vi "calc_rms.vi"(6 "Sampling Frequency [Hz]":dbl, 11 "Voltage [V]":dbl[](array[numeric])) -> (2 "Detected Frequency [Hz":dbl, 3 "RMS [V]":dbl)   [LabVIEW 2025, in "LabJackEKG.lvlib"]
uses:
  LabJackEKG.lvlib
  <vilib>/Analysis/2dsp.llb/Real FFT.vi
  <vilib>/Analysis/NI_AALPro.lvlib
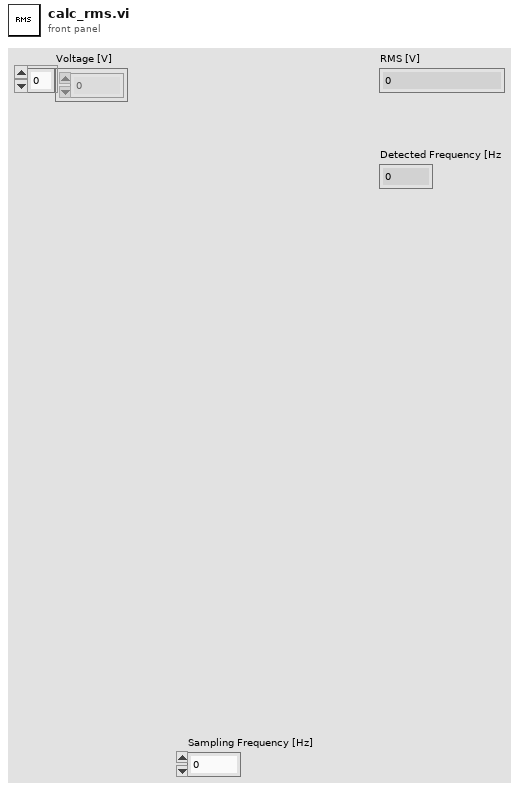
[diagram p1: front panel]
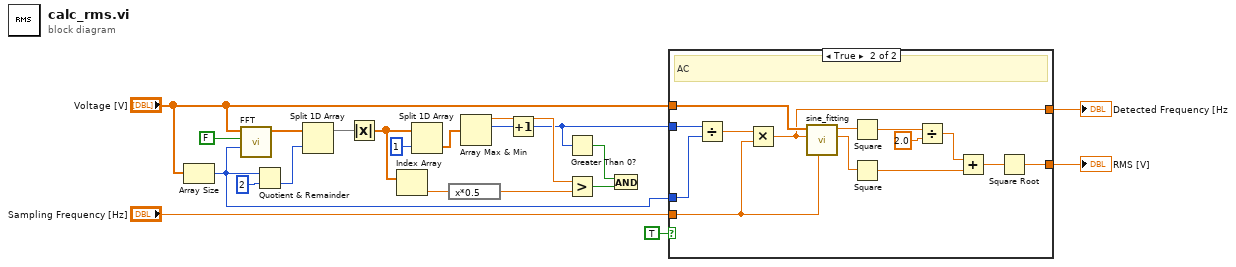
[diagram p0: block diagram]
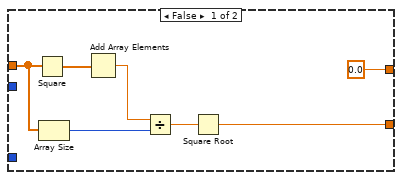
[diagram p2: hidden frame]
diagram:
  n1 = Array Size(array="Voltage [V]") -> (size(s)=w16:i32)
  n2 = call-poly <vilib>:"FFT.vi"("FFT size"=w16, "shift?"=FALSE, "X"="Voltage [V]") -> ("FFT {X}"=w8:cdb[])  [unwired: 7 in, 1 out]
  n3 = Quotient & Remainder(x=w16, y=2) -> (floor(x/y)=w10:i32)  [unwired: 1 out]
  n4 = Split 1D Array(array=w8, index=w10) -> (first subarray=w9:cdb[])  [unwired: 1 out]
  n5 = Absolute Value(x=w9) -> (abs(x)=w11:dbl[])
  n6 = Index Array(array=w11) -> (element=w13:dbl)  [unwired: 1 in]
  n7 = Split 1D Array(array=w11, index=1) -> (second subarray=w3:dbl[])  [unwired: 1 out]
  n8 = expression code="x*0.5"(w13) -> (w14:dbl)
  n9 = Array Max & Min(array=w3) -> (max value=w12:dbl, max index (indices)=w4:i32)  [unwired: 2 out]
  n10 = Increment(x=w4) -> (x+1=w1:i32)
  n11 = Greater Than 0?(x=w1) -> (x > 0?=w21:bool)
  n12 = Greater?(x=w12, y=w14) -> (0:w20:bool)
  n13 = And(x=w21, y=w20) -> ()  [unwired: 1 out]
  n14 = case shown="True" TRUE {
    tunnel: "Sampling Frequency [Hz]" -> [_ w38]
    tunnel: "Voltage [V]" -> [w24 w42]
    tunnel: w1 -> [_ w41]
    tunnel: w16 -> [_ w40]
    tunnel: [w25 w32] -> w17
    tunnel: [0.0 w29] -> w18
    frame False {
      n15 = Square(x=w24) -> (x^2=w28:dbl[])
      n16 = Array Size(array=w24) -> (size(s)=w23:i32)
      n17 = Add Array Elements(numeric array=w28) -> (sum=w27:dbl)
      n18 = Divide(x=w27, y=w23) -> (x/y=w26:dbl)
      n19 = Square Root(x=w26) -> (sqrt(x)=w25:dbl)
    }
    frame True {
      # "AC"
      n20 = Divide(x=w41, y=w40) -> (x/y=w39:dbl)
      n21 = Multiply(x=w39, y=w38) -> (x*y=w29:dbl)
      n22 = call "sine_fitting.vi"("Sampling Frequency [Hz]"=w38, "Frequency [Hz]"=w29, "RX data"=w42) -> ("DC Offset"=w36:dbl, "Amplidude"=w37:dbl)  [unwired: 7 in]
      n23 = Square(x=w37) -> (x^2=w34:dbl)
      n24 = Square(x=w36) -> (x^2=w30:dbl)
      n25 = Divide(x=w34, y=2.0) -> (x/y=w31:dbl)
      n26 = Add(x=w31, y=w30) -> (x+y=w33:dbl)
      n27 = Square Root(x=w33) -> (sqrt(x)=w32:dbl)
    }
  }
  "RMS [V]" <- w17
  "Detected Frequency [Hz" <- w18
